vi "Read MSG.vi"(8 "error in (no error)":errorcluster, 11 "Send MSG STEP in":refnum<class "Send MSG STEP.lvclass">) -> (0 "error out":errorcluster, 2 "Actor Framework:Message":refnum<class "Message.lvclass">, 3 "Send MSG STEP out":refnum<class "Send MSG STEP.lvclass">)   [LabVIEW 2014, in "Calibration.lvlib" / "Send MSG STEP.lvclass"]
uses:
  Send MSG STEP.lvclass
  <vilib>/ActorFramework/Message/Message.lvclass
  Send MSG STEP.lvclass/Send MSG STEP.ctl
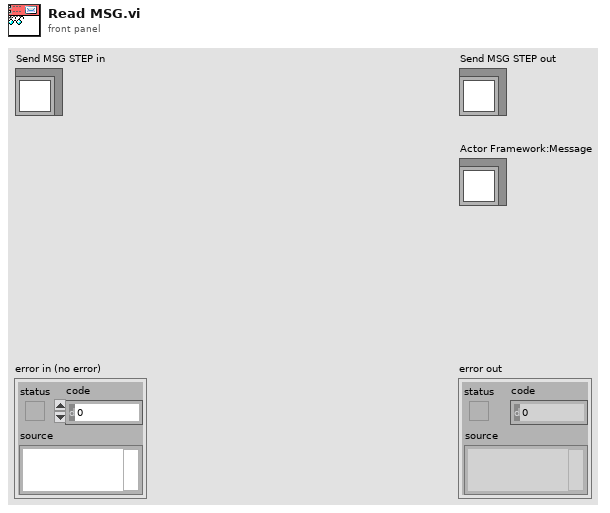
[diagram p1: front panel]
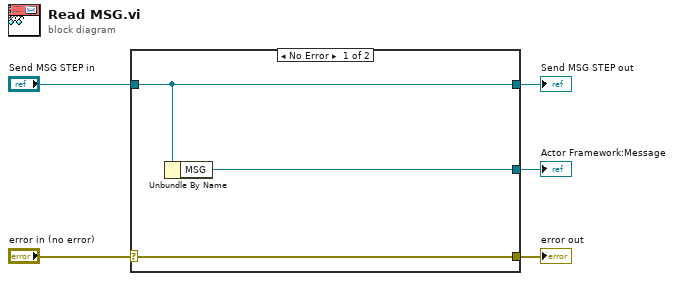
[diagram p0: block diagram]
diagram:
  n1 = case shown="No Error" "error in (no error)" {
    selector: "error in (no error)" -> [w8 w9]
    tunnel: [w8 w9] -> w4
    tunnel: [w7 w10] -> w2
    tunnel: "Send MSG STEP in" -> [w7 w10]
    tunnel: [w6 _] -> w1
    frame No Error {
      n2 = Unbundle By Name(w7) -> ("MSG"=w6:refnum<class "Message.lvclass">)
    }
    frame Error {
    }
  }
  "error out" <- w4
  "Send MSG STEP out" <- w2
  "Actor Framework:Message" <- w1
